vi "ZLIB Read Compressed File__ogtk.vi"(4 "permissions (0755)":i16=493 format="%.0o", 5 "overwrite (F)":bool, 6 "error in (no error)":errorcluster, 7 "uncompressed size":u32, 8 "target path":path, 9 "unzip Refnum":T1) -> (0 "error out":errorcluster, 3 "unzip Refnum out":T1)   [LabVIEW 2020]
doc: "Copies a file from a ZIP archive to disk."
uses:
  <userlib>/_OpenG.lib/lvzip/lvzlib.dll
  <userlib>/_OpenG.lib/lvzip/lvzip.llb/ZLIB Unzip Handle__ogtk.ctl
panel:
  # "Please visit http://www.OpenG.org to learn about the\nOpen Source LabVIEW software movement.\n\nNOTICE -- YOU MUST LEAVE THIS NOTICE IN PLACE.  PER THE TERMS OF THE LICENSE BELOW, YOU MAY SUBLICENSE THIS SOFTWARE \nIN ANY WAY THAT DOES NOT CONFLICT WITH THIS LICENSE.\n\n### BSD License (http://www.opensource.org/licenses/bsd-license.php) Begin ###\n \nCopyright (C) 2002-2004 Rolf Kalbermatter rolf.kalbermatter@citeng.com\nCopyright (C) 2002 Jim Kring jim@jimkring.com\n\nAll rights reserved.\n\nRedistribution and use in source and binary forms, with or without modification, are permitted provided that the following conditions are met:\n\n    * Redistributions of source code must retain the above copyright notice, this list of conditions and the following disclaimer.\n    * Redistributions in binary form must reproduce the above copyright notice, this list of conditions and the following disclaimer in the \n       documentation and/or other materials provided with the distribution.\n    * Neither the name of SciWare, James Kring, Inc., nor the names of its contributors may be used to endorse or promote products derived \n       from this software without specific prior written permission.\n\nTHIS SOFTWARE IS PROVIDED BY THE COPYRIGHT HOLDERS AND CONTRIBUTORS \"AS IS\" AND ANY EXPRESS OR IMPLIED WARRANTIES, \nINCLUDING, BUT NOT LIMITED TO, THE IMPLIED WARRANTIES OF MERCHANTABILITY AND FITNESS FOR A PARTICULAR PURPOSE ARE \nDISCLAIMED. IN NO EVENT SHALL THE COPYRIGHT OWNER OR CONTRIBUTORS BE LIABLE FOR ANY DIRECT, INDIRECT, INCIDENTAL,\n SPECIAL, EXEMPLARY, OR CONSEQUENTIAL DAMAGES (INCLUDING, BUT NOT LIMITED TO, PROCUREMENT OF SUBSTITUTE GOODS OR \nSERVICES; LOSS OF USE, DATA, OR PROFITS; OR BUSINESS INTERRUPTION) HOWEVER CAUSED AND ON ANY THEORY OF LIABILITY, \nWHETHER IN CONTRACT, STRICT LIABILITY, OR TORT (INCLUDING NEGLIGENCE OR OTHERWISE) ARISING IN ANY WAY OUT OF THE USE \nOF THIS SOFTWARE, EVEN IF ADVISED OF THE POSSIBILITY OF SUCH DAMAGE.\n\n### BSD License End ###"
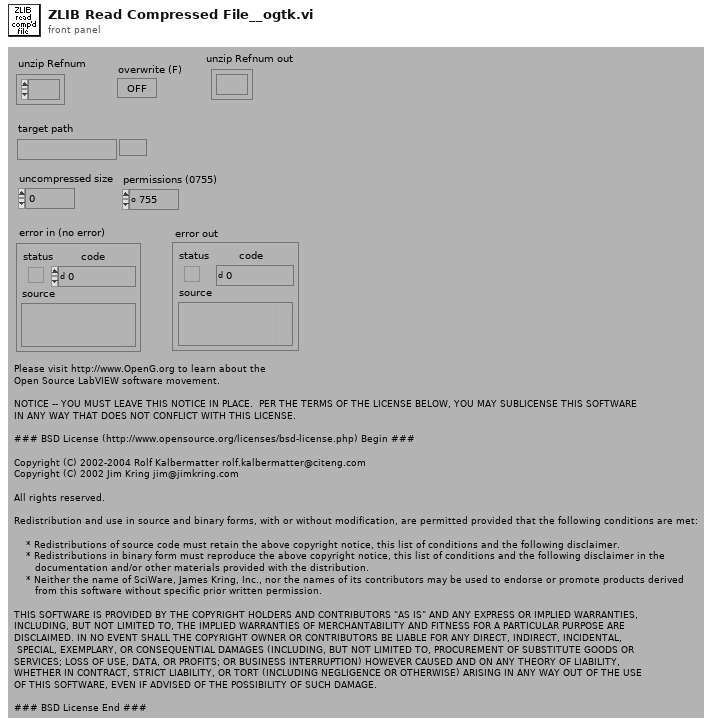
[diagram p1: front panel]
types:
  T1 = typedef "ZLIB Unzip Handle__ogtk.ctl" = refnum<k1>
  T2 = enum16{"open", "replace", "create", "open or create", "replace or create", "replace or create with confirmation"}
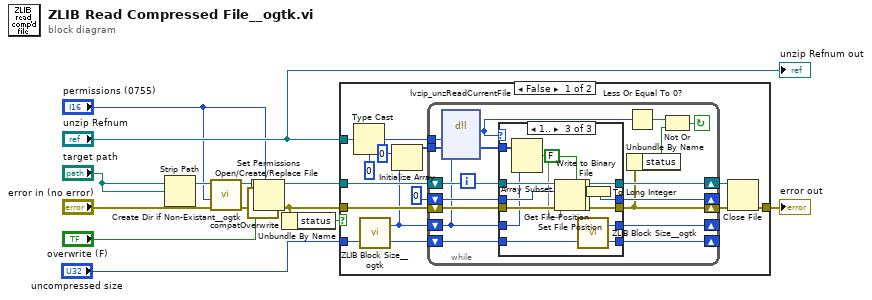
[diagram p0: block diagram]
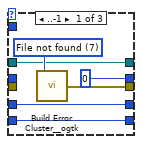
[diagram p2: hidden frame]
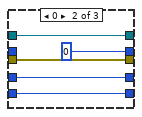
[diagram p3: hidden frame]
diagram:
  n1 = Strip Path(path="target path") -> (stripped path=w8:path)  [unwired: 1 out]
  n2 = call <userlib>:"Create Dir if Non-Existant__ogtk.vi"("error in (no error)"="error in (no error)", "permissions (0755)"="permissions (0755)", "Directory Path"=w8) -> ("error out"=w5:errorcluster)  [unwired: 6 in, 2 out]
  n3 = call <vilib>:"compatOverwrite.vi"("overwrite (F)"="overwrite (F)") -> ("overwrite?"=w1:T2)
  n4 = Open/Create/Replace File(file path (use dialog)="target path", error in=w5, operation (0:open)=w1) -> (refnum out=w11:refnum<file>, error out=w2:errorcluster)  [unwired: 3 in, 1 out]
  n5 = Set Permissions(7:"permissions (0755)", 8:w2, 11:"target path") -> (0:w12:errorcluster)  [unwired: 2 in, 1 out]
  n6 = Unbundle By Name(w12) -> ("status"=w13:bool)
  n7 = case shown="False" w13 {
    tunnel: w12 -> [w22 w75]
    tunnel: [w18 w75] -> w14
    tunnel: "unzip Refnum" -> [w27 _]
    tunnel: w11 -> [w23 _]
    tunnel: "uncompressed size" -> [w16 _]
    frame False {
      n8 = Type Cast(type=u32 0 ("unzFile"), x=w27) -> (*(type *) &x=w28:u32)
      n9 = call <userlib>:"ZLIB Block Size__ogtk.vi"("length in"=w16) -> ("length rem"=w15:u32, "block len"=w17:u32)  [unwired: 1 in]
      n10 = Initialize Array(u8 0 ("Element Data"), w17) -> (w24:u8[])
      n11 = while {
        shift-left: w17 -> [w29]
        shift-right: [w30] -> _
        shift-left: w15 -> [w32]
        shift-right: [w31] -> _
        shift-left: w23 -> [w39]
        shift-right: [w37] -> w20
        shift-left: w22 -> [w40]
        shift-right: [w33] -> w19
        shift-left: 0 ("offset") -> [w42]
        shift-right: [w41] -> _
        tunnel: w24 -> [w44]
        tunnel: w28 -> [w45]
        stop <- w34 continue-if-true
        n12 = dll-call lib="C:/Work/OpenG/opengtoolkit/lvzip/source/lvzlib.*" fn="lvzip_unzReadCurrentFile"("unzFile"=w45, "buffer"=w44, "size"=w29) -> (w43:i32, "buffer"=w38:u8[])  [unwired: 5 in, 2 out]
        n13 = case shown="1.." w43 {
          tunnel: w40 -> [_ w56 w74]
          tunnel: [w51 w56 w70] -> w33
          tunnel: w39 -> [w48 w54 w73]
          tunnel: w42 -> [_ _ w72]
          tunnel: [0 ("offset") 0 ("offset") w71] -> w41
          tunnel: [w48 w54 w69] -> w37
          tunnel: w38 -> [_ _ w64]
          tunnel: w32 -> [w46 w52 w68]
          tunnel: [w46 w52 w67] -> w31
          tunnel: [w47 w53 w66] -> w30
          tunnel: w29 -> [w47 w53 w65]
          frame ..-1 {
            w50 = 7 items=["No error", "Argument error", "Memory is full", "Out of zone", "End of file", "File already open", "Generic file I/O error", "File not found", "File permission error", "Disk is full", "Duplicate path", "Too many files open", "System feature not enabled", "Resource file not found", "Cannot add resource", "Resource not found", "Image not found", "Image memory error", "Pen does not exist", "Config type invalid", "Config token not found", "Config parse error", "Config memory error", "Bad external code format", "Bad external code offset", "External code not present", "Null window", "Destroy window error", "Null menu", "Print aborted", "Bad print record", "Print driver error", "Windows error during printing", "Memory error during printing", "Print dialog error", "Generic print error", "Invalid device refnum", "Device not found", "Device parameter error", "Device unit error", "Cannot open device", "Device call aborted", "Generic error", "Cancelled by user", "Object ID too low", "Object ID too high", "Object not in heap", "Unknown heap", "Unknown object (invalid DefProc)", "Unknown object (DefProc not in table)", "Message out of range", "Invalid (null) method", "Unknown message", "Manager call not supported", "Bad address", "Network operation in progress", "Network operation timed out", "Connection is busy", "Network attribute not supported", "Network error", "Address in use", "System out of memory", "Connection aborted", "Connection refused", "Not connected", "Already connected", "Connection closed", "Initialization error (interapplication manager)", "Bad occurrence", "Wait on unbound occurrence handler", "Occurrence queue overflow", "Datalog type conflict", "Unused", "Unrecognized type (interapplication manager)", "Memory corrupt", "Failed to make temporary DLL", "Old CIN version", "Drag socket not found", "Failed to load drop-object", "Failed to register OLE object", "Failed to release OLE object", "Format specifier type mismatch", "Unknown format specifier", "Too few format specifiers", "Too many format specifiers", "Scan failed", "Newer CIN version", "Error converting to variant", "Runtime menu error", "Password tampered", "Variant attribute not found", "Incompatible variant data type", "Event data is not available", "Event Store is not present", "Occurrence is not found", "Event Queue is not created", "Event info is not available", "Refnum passed is NULL", "Error retrieving Class GUID", "Error retrieving CoClass GUID", "Error retrieving TypeLib GUID.", "Bad built application magic bytes.", "Specific driver is different from the specific driver associated with the Logical Name.", "There is no session opened to the class driver.", "Max Error", "MAX - Error with config objects", "MAX - Error loading configuration", "MAX - Group not supported"]
            n14 = call <userlib>:"Build Error Cluster__ogtk.vi"("code"=w50) -> ("error out"=w51:errorcluster)  [unwired: 1 in]
          }
          frame 0 {
          }
          frame 1.. {
            n15 = Array Subset(array=w64, length=w65) -> (w63:u8[])  [unwired: 1 in]
            n16 = Set File Position(offset (in bytes) (0)=w72, refnum=w73, error in=w74) -> (refnum out=w62:refnum<file>, error out=w61:errorcluster)  [unwired: 1 in]
            n17 = Write to Binary File(file (use dialog)=w62, data=w63, error in=w61, 5:FALSE ("prepend array or string size? (T)")) -> (refnum out=w60:refnum<file>, error out=w59:errorcluster)  [unwired: 2 in, 1 out]
            n18 = Get File Position(4:w59, 7:w60) -> (0:w70:errorcluster, 2:w58:i64, 3:w69:refnum<file>)
            n19 = call <userlib>:"ZLIB Block Size__ogtk.vi"("length in"=w68) -> ("length rem"=w67:u32, "block len"=w66:u32)  [unwired: 1 in]
            n20 = To Long Integer(number=w58) -> (32bit integer=w71:i32)
          }
        }
        n21 = Less Or Equal To 0?(x=w43) -> (x <= 0?=w35:bool)
        n22 = Unbundle By Name(w33) -> ("status"=w36:bool)
        n23 = Not Or(1:w36, 2:w35) -> (0:w34:bool)
      }
      n24 = Close File(refnum=w20, error in=w19) -> (error out=w18:errorcluster)  [unwired: 1 out]
    }
    frame True {
    }
  }
  "error out" <- w14
  "unzip Refnum out" <- "unzip Refnum"
